vi "MRate Decimation (Host).vi"() -> ()   [LabVIEW 2023]
uses:
  <vilib>/rvi/interface/nirviOpenFPGA/nirviOpenFPGA.xnode
  <vilib>/rvi/interface/nirviMethod/nirviMethod.xnode
  <vilib>/rvi/interface/nirviCloseFPGA/nirviCloseFPGA.xnode
  <vilib>/addons/Digital Filter Design/NI_DigFilterLicensed.lvlib
  <vilib>/addons/Digital Filter Design/FXPMRateSim.llb/DFD FXP MRate Postprocessing (I32, 1Ch).vi
  <vilib>/addons/Digital Filter Design/FilterLib.llb/DFD Load MRate Filter from File.vi
  <vilib>/rvi/errors/niLvFpgaMergeErrorWithErrorCode.vi
  FPGA Bitfiles/MRateDecimation_FPGATarget_MRateDecimation(_PpvkXnERzuE.lvbitx
  MRate Decimation (FPGA).vi
  <vilib>/userdefined/High Color/nirio_resource_hc.ctl
panel:
  out "error out":errorcluster
  in  "Resource Name":T1="RIO0::INSTR"
  in  "stop":bool
  out "Filtered Signal":dbl[](graph)
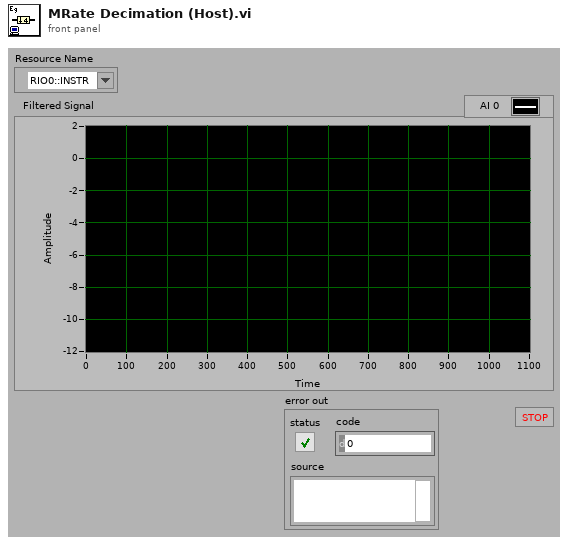
[diagram p1: front panel]
types:
  T1 = typedef "nirio_resource_hc.ctl" = tag
  T2 = typedef "NI_DigFilterLicensed.lvlib/DFD Multirate Filter Obj.ctl" = cluster{"mMRate_Structure":enum16{"CIC", "FIR", "IIR", "Lattice"}, "mMRate_Mode":T3, "mMRate_Factor":i32, "mMRate_FIRParams":cluster{"mMRate_FIR_H":dbl[], "mMRate_FIR_IsNyquist?":bool, "mMRate_FIR_IsSymmetric?":bool}, "mMRate_CICParams":cluster{"mMRate_CIC_#Stage":i32, "mMRate_CIC_Lag":i32, "mMRate_CIC_Type":enum16{"Lowpass", "Highpass"}}, "mMRate_Order":i32, "mMRate_Version":string, "mMRate_Comments":string, "mMRate_RationalFactor":cluster{"mMRate_L":i32, "mMRate_M":i32}, "mMRate_Fs":dbl, "mMRate_Quantized?":bool, "mMRate_QFilterGain":dbl, "mMRate_CoefWl":i16, "mMRate_Scaling":cluster{"mMRate_ScaleByPowerOf2?":bool, "mMRate_ScaleType":T4}, "mMRate_InputWl":i16, "mMRate_OutputWl":i16, "mMRate_OutputMode":T5, "mMRate_MultMode":T6, "mMRate_BitPruning":bool, "mMRate_GainWl":i16, "mMRate_OutputFwl":i16, "mMRate_SumIwl":i16, "mMRate_InputIwl ":i16, "mMRate_SumWl":i16, "mMRate_CoefIwl":i16}
  T3 = typedef "NI_DigFilterLicensed.lvlib/DFD Multirate Mode.ctl" = i16
  T4 = typedef "NI_DigFilterLicensed.lvlib/DFD Coef Norm Type.ctl" = enum16{"No Norm", "Time Domain 1-Norm", "Time Domain 2-Norm", "Time Domain Inf-Norm"}
  T5 = typedef "NI_DigFilterLicensed.lvlib/DFD Round-off Mode.ctl" = enum16{"Nearest", "Truncation"}
  T6 = typedef "NI_DigFilterLicensed.lvlib/DFD FXP MRate Multiply Mode.ctl" = enum16{"Truncated", "Full"}
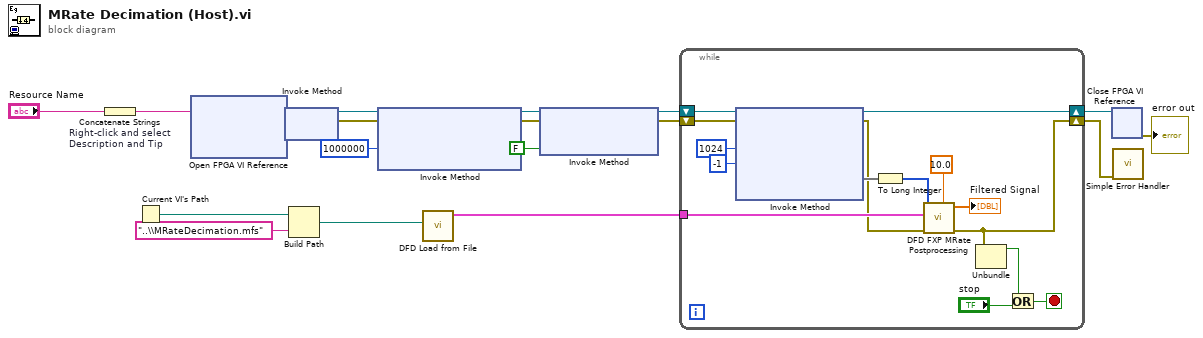
[diagram p0: block diagram]
diagram:
  n1 = Concatenate Strings "Right-click and select Description and Tip"("Resource Name") -> (w3:string)
  n2 = Current VI's Path() -> (path=w7:path)
  n3 = xnode "Open FPGA VI Reference"("resource name"=w3) -> ("FPGA VI Reference Out"=w19:refnum<k20>, "error out"=w18:errorcluster)  [unwired: 1 in]
  n4 = xnode "Invoke Method"("FPGA VI Reference In"=w19, "error in"=w18) -> ("FPGA VI Reference Out"=w17:refnum<k20>, "error out"=w16:errorcluster)
  n5 = Build Path(base path=w7, name or relative path="..\\MRateDecimation.mfs") -> (appended path=w5:path)
  n6 = xnode "Invoke Method"("FPGA VI Reference In"=w17, "error in"=w16, "Requested Depth"=u32 1000000 ("Depth")) -> ("FPGA VI Reference Out"=w14:refnum<k20>, "error out"=w13:errorcluster)  [unwired: 1 out]
  n7 = call-poly <vilib>:"DFD Load from File.vi"("file path in"=w5) -> ("multirate filter out"=w4:T2)  [unwired: 1 in, 9 out]
  n8 = xnode "Invoke Method"("FPGA VI Reference In"=w14, "error in"=w13, "Wait Until Done (F)"=FALSE) -> ("FPGA VI Reference Out"=w12:refnum<k20>, "error out"=w11:errorcluster)
  n9 = while {
    shift-right: [w23] -> w9
    shift-left: w11 -> [w33]
    tunnel: w4 -> [w28]
    shift-right: [w24] -> w10
    shift-left: w12 -> [w34]
    stop <- w20 stop-if-true
    n10 = xnode "Invoke Method"("FPGA VI Reference In"=w34, "error in"=w33, "Number of Elements"=u32 1024, "Timeout (ms)"=-1) -> ("FPGA VI Reference Out"=w24:refnum<k20>, "error out"=w27:errorcluster, "Data"=w30:void[])  [unwired: 1 out]
    n11 = To Long Integer(number=w30) -> (32bit integer=w29:i32[])
    n12 = call-poly <vilib>:"DFD FXP MRate Postprocessing.vi"("input range"=10.0, "error in (no error)"=w27, "multirate filter"=w28, "signal in"=w29) -> ("error out"=w23:errorcluster, "signal out"=→"Filtered Signal":dbl[])  [unwired: 1 in, 5 out]
    n13 = Unbundle(w23) -> ("status"=w21:bool)  [unwired: 2 out]
    n14 = Or(x=w21, y="stop") -> (x .or. y?=w20:bool)
  }
  n15 = xnode "Close FPGA VI Reference"("FPGA VI Reference In"=w10) -> ("error out"=→"error out":errorcluster)  [unwired: 1 in]
  n16 = call <vilib>:"Simple Error Handler.vi"("error in (no error)"=w9) -> ()  [unwired: 1 in, 8 out]
